vi "LCD Configure 4-bit.vi"(8 "Error In":errorcluster, 10 "LCD Pin Config 4 Bit":T1={"RS"=12, "RW"=255, "Enable"=11, "D4"=5, "D5"=4, "D6"=3, "D7"=2}, 11 "ChipKit Resource":T2={"COM Port"="", "Board Type"=enum."ChipKit Uno32", "Connection Type"=enum."USB / Serial", "Baud Rate (115200)"=0, "Bytes Per Packet (15)"=15, "DI Port Num Pins"=0, "DO Port Num Pins"=0}) -> (0 "Error Out":errorcluster, 3 "ChipKit Resource":T2={"COM Port"="", "Board Type"=enum."ChipKit Uno32", "Connection Type"=enum."USB / Serial", "Baud Rate (115200)"=0, "Bytes Per Packet (15)"=15, "DI Port Num Pins"=0, "DO Port Num Pins"=0})   [LabVIEW 2011, in "LabVIEW Interface for ChipKit.lvlib"]
doc: "Configures the LCD according to the input pin configuration. A 4-bit setup configuration can be selected. If the RW pin is disconnected, or connected to ground, set the RW pin to 255."
uses:
  LabVIEW Interface for ChipKit.lvlib
  Private/Type Defs/Chipkit Resource.ctl
  Private/Type Defs/Board Type.ctl
  Private/Type Defs/Connection Type.ctl
  Private/Type Defs/LCD Pin Config 4-bit.ctl
  Private/Type Defs/Command.ctl
  Private/Type Defs/Pin Mode.ctl
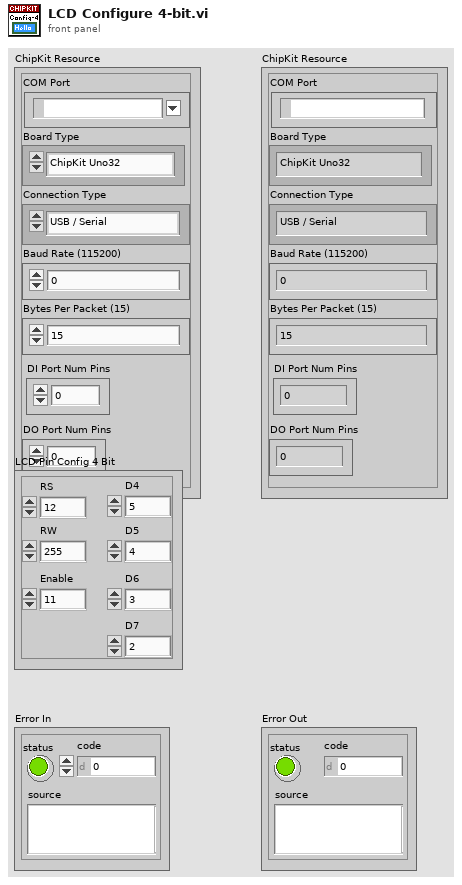
[diagram p1: front panel]
types:
  T1 = typedef "LabVIEW Interface for ChipKit.lvlib/LCD Pin Config 4-bit.ctl" = cluster{"RS":u8, "RW":u8, "Enable":u8, "D4":u8, "D5":u8, "D6":u8, "D7":u8}
  T2 = typedef "LabVIEW Interface for ChipKit.lvlib/Chipkit Resource.ctl" = cluster{"COM Port":refnum<visa-resource-name>, "Board Type":T3, "Connection Type":T4, "Baud Rate (115200)":u32, "Bytes Per Packet (15)":u32, "DI Port Num Pins":i32, "DO Port Num Pins":i32}
  T3 = typedef "LabVIEW Interface for ChipKit.lvlib/Board Type.ctl" = enum16{"ChipKit uC32", "ChipKit Uno32", "ChipKit Max32"}
  T4 = typedef "LabVIEW Interface for ChipKit.lvlib/Connection Type.ctl" = enum8{"USB / Serial", "XBEE", "BlueSmirf (Bluetooth)"}
  T5 = typedef "LabVIEW Interface for ChipKit.lvlib/Pin Mode.ctl" = enum16{"Input", "Output"}
  T6 = typedef "LabVIEW Interface for ChipKit.lvlib/Command.ctl" = enum8{"setArduinoMode", "flushSerial", "setPinMode", "digitalWritePin", "digitalWritePort", "tone", "digitalReadPin", "digitalReadPort", "analogReadPin", "analogReadPort", "pwmWritePin", "pwmWritePort", "sevenSegment_Configure", "sevenSegment_Write", "I2C Init", "I2C Write", "I2C Read", "SPI Init", "SPI Set Bit Order", "SPI Set Clock Divider", "SPI Set Data Mode", "SPI Send / Receive", "SPI Close", "Servo Set Num Servos", "Servo Config Servo", "Servo Write Angle", "Servo Read Angle", "Servo Write Pulse Width", "Servo Read Pulse Width", "Servo Detach", "LCD Init", "LCD Set Size", "LCD Set Cursor Mode", "LCD Clear", "LCD Set Cursor Position", "LCD Print", "LCD Display Power", "LCD Scroll Display", "LCD Autoscroll", "LCD Print Direction", "LCD Create Custom Char", "LCD Print Custom Char", "contAcqOn", "contAcqOff", "getFirmwareVersion", "FiniteSampleStart", "NA", "NA2", "Conifg Stepper", "Stepper Write", "Stepper Detach", "Stepper Steps To Go", "Config DO Port", "Config DI Port", "UART2 Open", "UART2 Write", "UART2 Bytes Available", "UART2 Read"}
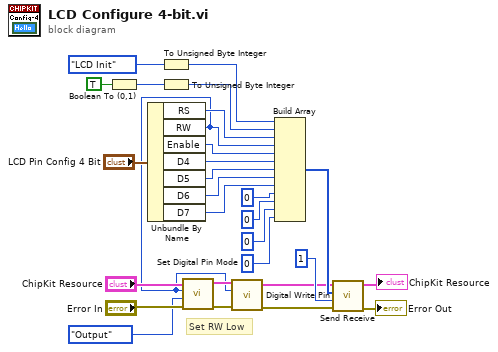
[diagram p0: block diagram]
diagram:
  # "Set RW Low"
  n1 = Boolean To (0,1)(Boolean=TRUE) -> (0, 1=w16:i16)
  n2 = Unbundle By Name("LCD Pin Config 4 Bit") -> ("RS"=w17:u8, "RW"=w2:u8, "Enable"=w18:u8, "D4"=w19:u8, "D5"=w20:u8, "D6"=w21:u8, "D7"=w22:u8)
  n3 = To Unsigned Byte Integer(number=Command."LCD Init" ("Command")) -> (unsigned 8bit integer=w24:u8)
  n4 = To Unsigned Byte Integer(number=w16) -> (unsigned 8bit integer=w15:u8)
  n5 = call "Set Digital Pin Mode.vi"("Error In"="Error In", "Pin Mode (Input)"=Pin_Mode."Output", "Digital I/O Pin"=w2, "Arduino Resource"="ChipKit Resource") -> ("Error Out"=w8:errorcluster, "Arduino Resource"=w7:T2)  [unwired: 6 in]
  n6 = call "Digital Write Pin.vi"("Error In"=w8, "Digital I/O Pin (2)"=w2, "ChipKit Resource"=w7) -> ("Error Out"=w4:errorcluster, "ChipKit Resource"=w3:T2)  [unwired: 7 in]
  n7 = Build Array(w24, w15, w17, w2, w18, w19, w20, w21, w22, u8 0 ("element"), u8 0 ("element"), u8 0 ("element"), u8 0 ("element")) -> (w25:u8[])
  n8 = call "Send Receive.vi"("Error In"=w4, "Bytes To Read (0)"=u8 1, "Data"=w25, "ChipKit Resource"=w3) -> ("Error Out"=→"Error Out":errorcluster, "ChipKit Resource"=→"ChipKit Resource":T2)  [unwired: 5 in, 1 out]
